vi "ProccessTableToTreePlantUML.vi"() -> ()   [LabVIEW 2020]
uses:
  <vilib>/regexp/Match Regular Expression.xnode
panel:
  out "format string":string
  in  "Input":string="| 309 | Critical Speed Limit | Alarm | The critical speed limit was violated | Reset alarm |\n| 310 | Positive Software Limit | Alarm | The positive software limit is overcomed | Disable the software limit using the settings and Reset alarm |\n| 311 | Negative Software Limit | Alarm | The negative software limit is overcomed | Disable the software limit using the settings and Reset alarm |\n| 312 | Azimuth Cable Wrap Safety | Alarm | A safety issue has ocurred in the azimuth cable wrap module | Check the safety cause and reset it if necessary then Reset alarm |\n| 314 | Critical Azimuth Deviation Limit | Alarm | The maximum allowed deviation between azimuth position and azimuth cable wrap position was overcomed | Center the ACW to the Azimuth position and Reset alarm |\n| 315 | Main Cabinet Off | Alarm | A fault ocurred at the Main Cabinet that is going to power off the cabinet. | Reset the alarm from the main temperature cabinet and then Reset alarm |\n| 370 | Bosch Power Supply Off | Alarm | The bosch power supply is off , therefore the systems that use the bosch drives cannot be used. | Check that the bosch power supply is on then Reset alarm |"
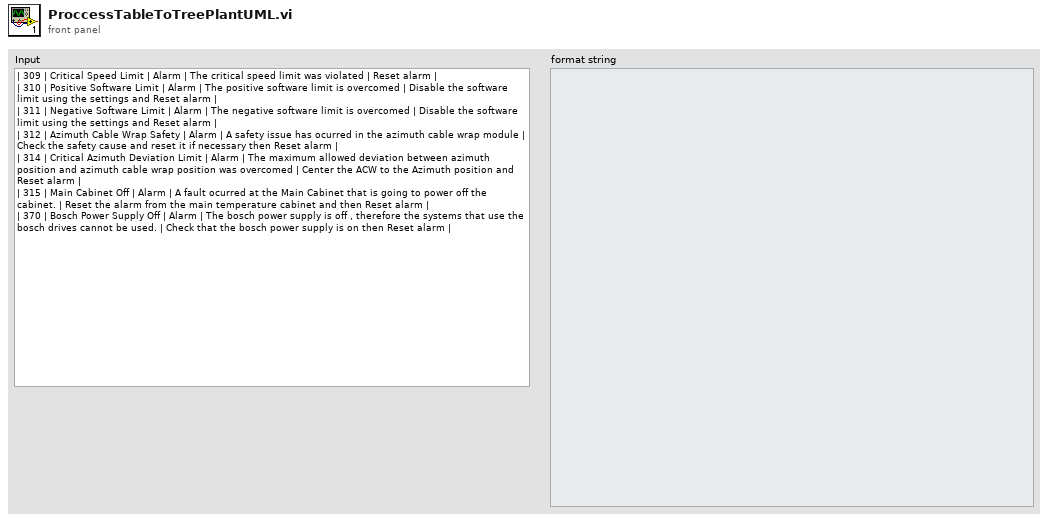
[diagram p1: front panel]
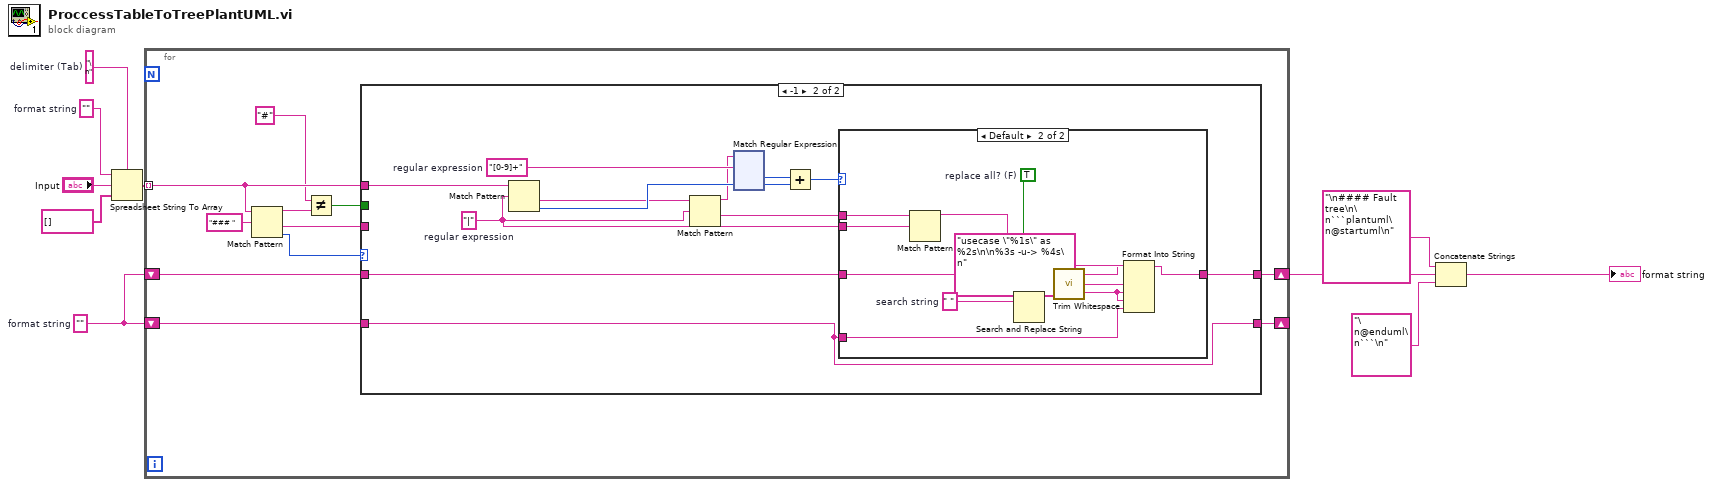
[diagram p0: block diagram]
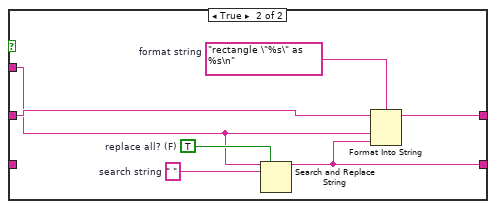
[diagram p3: hidden frame]
diagram:
  w3 = ""  # format string
  w7 = "\n"  # delimiter (Tab)
  w8 = ""  # format string
  n1 = Spreadsheet String To Array(delimiter (Tab)=w7, format string=w8, spreadsheet string="Input", array type (2D Dbl)=string[] []) -> (array=w6:string[])
  n2 = for {
    tunnel: w6 -> [w19] mode=indexing
    shift-right: [w20] -> w5
    shift-left: w3 -> [w21]
    shift-right: [w12] -> _
    shift-left: w3 -> [w11]
    n3 = Match Pattern(string=w19, regular expression="### ") -> (before substring=w16:string, after substring=w13:string, offset past match=w17:i32)  [unwired: 1 in, 1 out]
    n4 = Not Equal?(x="#", y=w16) -> (x != y?=w14:bool)
    n5 = case shown="-1" w17 {
      tunnel: w19 -> [_ w48]
      tunnel: w21 -> [w26 w46]
      tunnel: [w25 w45] -> w20
      tunnel: w14 -> [w27 _]
      tunnel: w13 -> [w24 _]
      tunnel: [w23 w37] -> w12
      tunnel: w11 -> [w22 w37]
      frame Default {
        n6 = case shown="False" w27 {
          tunnel: w26 -> [w29 w33]
          tunnel: [w29 w31] -> w25
          tunnel: w24 -> [_ w32]
          tunnel: [w28 w30] -> w23
          tunnel: w22 -> [w28 _]
          frame False {
          }
          frame True {
            w36 = TRUE  # replace all? (F)
            w34 = "rectangle \"%s\" as %s\n"  # format string
            w35 = " "  # search string
            n7 = Search and Replace String(replace all?=w36, input string=w32, search string=w35) -> (result string=w30:string)  [unwired: 5 in, 3 out]
            n8 = Format Into String(format string=w34, initial string=w33, w32, w30) -> (resulting string=w31:string)  [unwired: 1 in, 1 out]
          }
        }
      }
      frame -1 {
        w44 = "[0-9]+"  # regular expression
        w47 = "|"  # regular expression
        n9 = Match Pattern(string=w48, regular expression=w47) -> (after substring=w40:string, offset past match=w42:i32)  [unwired: 1 in, 2 out]
        n10 = Match Pattern(string=w40, regular expression=w47) -> (before substring=w38:string, after substring=w39:string)  [unwired: 1 in, 2 out]
        n11 = xnode "Match Regular Expression"("input string"=w38, "regular expression"=w44) -> ("offset past match"=w43:i32)  [unwired: 4 in, 4 out]
        n12 = Add(x=w43, y=w42) -> (x+y=w41:i32)
        n13 = case shown="Default" w41 {
          tunnel: w47 -> [_ w174]
          tunnel: w46 -> [w163 w170]
          tunnel: [w163 w169] -> w45
          tunnel: w39 -> [_ w167]
          tunnel: w37 -> [_ w165]
          frame ..0 {
          }
          frame Default {
            w168 = TRUE  # replace all? (F)
            w173 = " "  # search string
            n14 = Match Pattern(string=w167, regular expression=w174) -> (before substring=w171:string)  [unwired: 1 in, 3 out]
            n15 = Search and Replace String(replace all?=w168, input string=w171, search string=w173) -> (result string=w164:string)  [unwired: 5 in, 3 out]
            n16 = call <vilib>:"Trim Whitespace.vi"("string"=w171) -> ("trimmed string"=w166:string)  [unwired: 1 in]
            n17 = Format Into String(format string="usecase \"%1s\" as %2s\n\n%3s -u-> %4s\n", initial string=w170, w166, w164, w164, w165) -> (resulting string=w169:string)  [unwired: 1 in, 1 out]
          }
        }
      }
    }
  }
  n18 = Concatenate Strings("\n#### Fault tree\n\n```plantuml\n@startuml\n", w5, "\n@enduml\n```\n") -> (→"format string":string)
